vi "Callback Ex.vi"   [LabVIEW 2020]
uses:
  Callback Producer/Callback Producer.lvclass
  Callback Consumer/Callback Consumer.lvclass
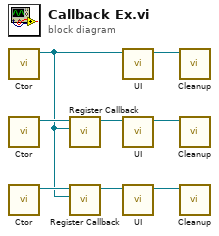
[diagram p0: block diagram]
diagram:
  n1 = call "Ctor.vi"() -> ("Callback Producer out"=w4:refnum<class "Callback Producer.lvclass">)  [unwired: 10 in, 1 out]
  n2 = call "Ctor.vi"() -> ("Callback Consumer out"=w8:refnum<class "Callback Consumer.lvclass">)  [unwired: 10 in, 1 out]
  n3 = call "Ctor.vi"() -> ("Callback Consumer out"=w7:refnum<class "Callback Consumer.lvclass">)  [unwired: 10 in, 1 out]
  n4 = call "Register Callback.vi"("Producer"=w4, "Callback Consumer in"=w8) -> ("Callback Consumer out"=w6:refnum<class "Callback Consumer.lvclass">)  [unwired: 8 in, 1 out]
  n5 = call "Register Callback.vi"("Producer"=w4, "Callback Consumer in"=w7) -> ("Callback Consumer out"=w5:refnum<class "Callback Consumer.lvclass">)  [unwired: 8 in, 1 out]
  n6 = call "UI.vi"("Callback Producer in"=w4) -> ("Callback Producer out"=w3:refnum<class "Callback Producer.lvclass">)  [unwired: 9 in, 1 out]
  n7 = call "UI.vi"("Callback Consumer in"=w6) -> ("Callback Consumer out"=w2:refnum<class "Callback Consumer.lvclass">)  [unwired: 9 in, 1 out]
  n8 = call "UI.vi"("Callback Consumer in"=w5) -> ("Callback Consumer out"=w1:refnum<class "Callback Consumer.lvclass">)  [unwired: 9 in, 1 out]
  n9 = call "Cleanup.vi"("Callback Producer in"=w3) -> ()  [unwired: 10 in, 1 out]
  n10 = call "Cleanup.vi"("Callback Consumer in"=w2) -> ()  [unwired: 10 in, 1 out]
  n11 = call "Cleanup.vi"("Callback Consumer in"=w1) -> ()  [unwired: 10 in, 1 out]
